vi "ProvaAdquisicioDadesYoctopuce.vi"(10 "Temperature name":string="THRMCPL1-204875.temperature1") -> (0 "error out":errorcluster)   [LabVIEW 2017]
panel:
  in  "AssaigActiu":bool
  in  "stop":bool
  out "error msg":string
  out "hardware name":string
  out "isOnline 2":bool
  out "Temp":dbl
  out "appended array":sgl[](array[numeric])
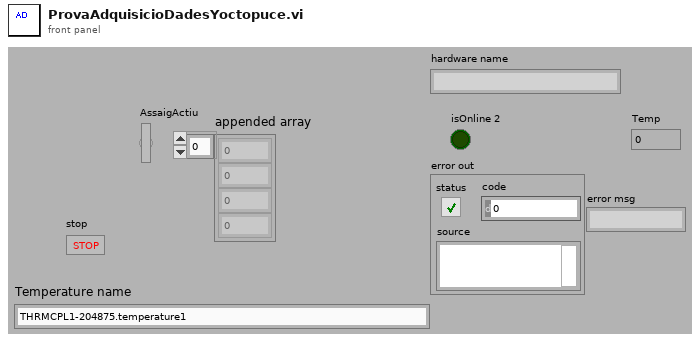
[diagram p1: front panel]
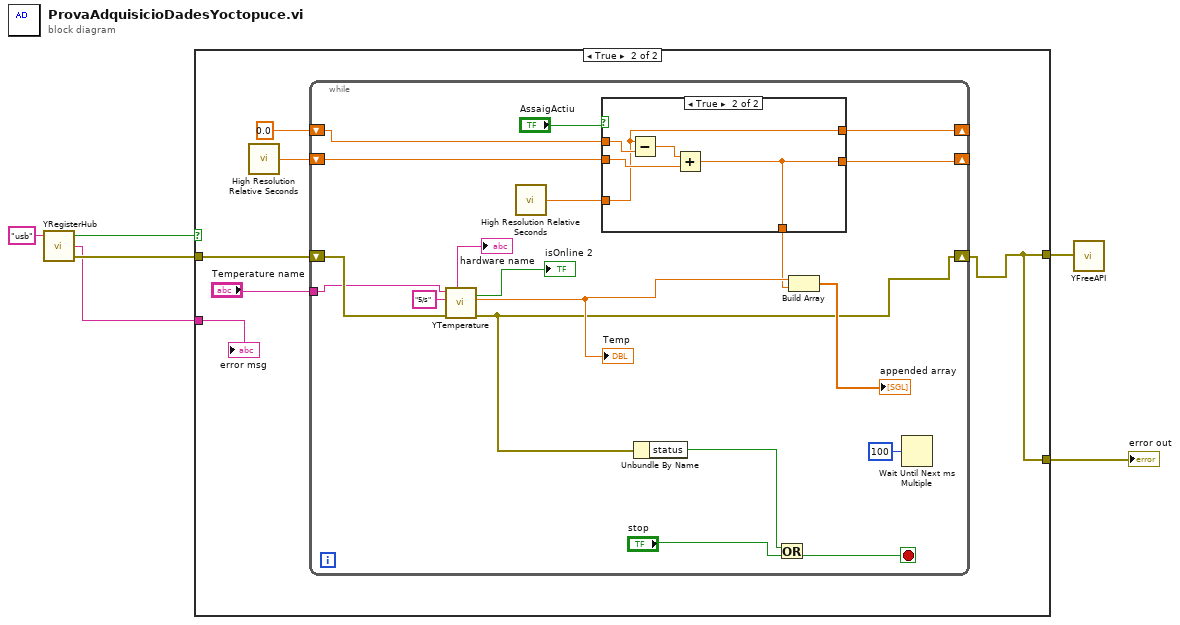
[diagram p0: block diagram]
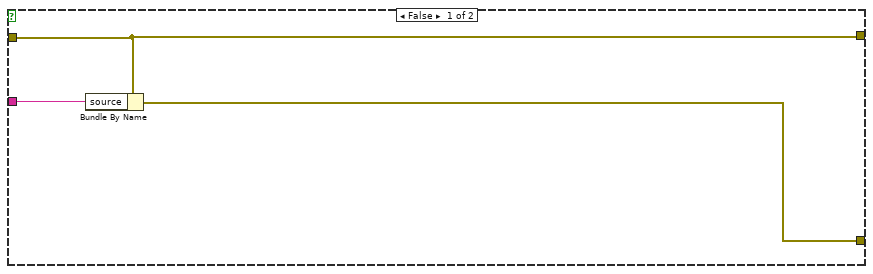
[diagram p2: hidden frame]
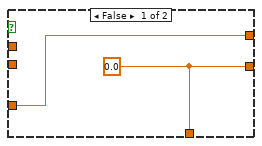
[diagram p3: hidden frame]
diagram:
  n1 = call "YRegisterHub.vi"("url"="usb") -> ("error out"=w6:errorcluster, "error msg"=w1:string, "success"=w4:bool)  [unwired: 2 in]
  n2 = case shown="True" w4 {
    tunnel: w6 -> [w8 w15]
    tunnel: [w8 w14] -> w3
    tunnel: [w7 w14] -> w2
    tunnel: w1 -> [w9 w10]
    frame False {
      n3 = Bundle By Name(cluster=w8, "source"=w9) -> (w7:errorcluster)
    }
    frame True {
      n4 = call <vilib>:"High Resolution Relative Seconds.vi"() -> ("relative seconds"=w12:dbl)
      n5 = while {
        shift-right: [w21] -> w14
        shift-left: w15 -> [w24]
        shift-right: [w25] -> _
        shift-left: 0.0 ("relative seconds") -> [w28]
        shift-right: [w26] -> _
        shift-left: w12 -> [w30]
        tunnel: "Temperature name" -> [w16]
        stop <- w31 stop-if-true
        n6 = call "YTemperature.vi"("error in (no error)"=w24, "reportFrequency in"="5/s", "Temperature name"=w16) -> ("error out"=w21:errorcluster, "currentValue out"=w34:dbl, "isOnline"=→"isOnline 2":bool, "hardware name"=→"hardware name":string)  [unwired: 3 in, 2 out]
        "Temp" <- w34
        n7 = call <vilib>:"High Resolution Relative Seconds.vi"() -> ("relative seconds"=w29:dbl)
        n8 = case shown="True" "AssaigActiu" {
          tunnel: w30 -> [_ w40]
          tunnel: w29 -> [w36 w37]
          tunnel: w28 -> [_ w39]
          tunnel: [w35 w38] -> w27
          tunnel: [w35 w38] -> w26
          tunnel: [w36 w37] -> w25
          frame False {
            w35 = 0.0
          }
          frame True {
            n9 = Subtract(x=w37, y=w39) -> (x-y=w41:dbl)
            n10 = Add(x=w41, y=w40) -> (x+y=w38:dbl)
          }
        }
        n11 = Unbundle By Name(w21) -> ("status"=w20:bool)
        n12 = Or(x=w20, y="stop") -> (x .or. y?=w31:bool)
        n13 = Build Array(w34, w27) -> (→"appended array":dbl[])
        n14 = Wait Until Next ms Multiple(millisecond multiple=u32 100) -> ()  [unwired: 1 out]
      }
      "error msg" <- w10
    }
  }
  "error out" <- w2
  n15 = call "YFreeAPI.vi"("error in (no error)"=w3) -> ()  [unwired: 1 out]
